vi "1.1 - Building a linear light detector using a biased photodiode.vi"() -> ()   [LabVIEW 2017]
panel:
  out "output array":dbl[](graph)
  in  "stop":bool
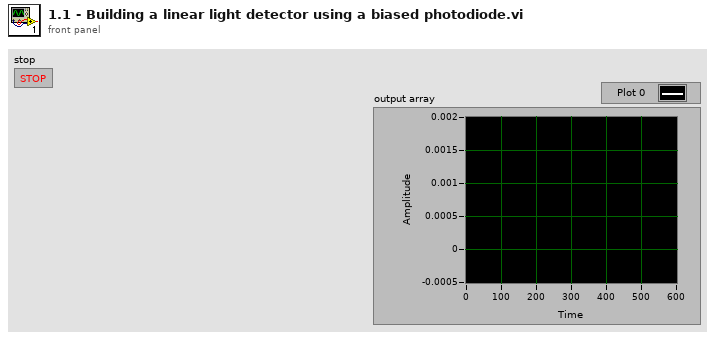
[diagram p1: front panel]
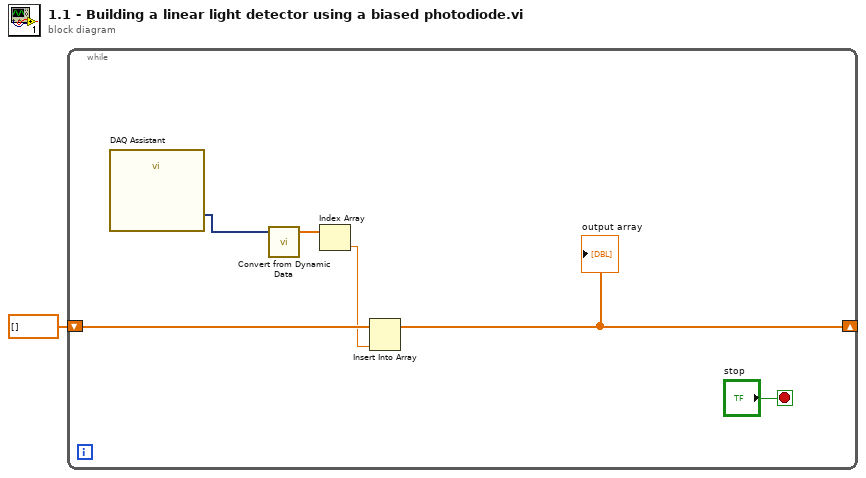
[diagram p0: block diagram]
diagram:
  n1 = while {
    shift-right: [w6] -> _
    shift-left: dbl[] [] -> [w5]
    stop <- "stop" stop-if-true
    n2 = call "DAQ Assistant"() -> ("data"=w3:dynamicdata)  [unwired: 17 in, 2 out]
    n3 = call "Convert from Dynamic Data"("Dynamic Data Type"=w3) -> ("Array"=w4:dbl[])  [unwired: 3 in]
    n4 = Index Array(array=w4) -> (element=w2:dbl)  [unwired: 1 in]
    n5 = Insert Into Array(array=w5, new element=w2) -> (w6:dbl[])  [unwired: 1 in]
    "output array" <- w6
  }
